vi "Get Bytes.vi"(11 "IMessagePackObject in":refnum<class "IMessagePackObject.lvclass">) -> (2 "Array":u8[](array[numeric]), 3 "IMessagePackObject out":refnum<class "IMessagePackObject.lvclass">)   [LabVIEW 2020, in "wamplv.lvlib" / "IMessagePackObject.lvclass"]
uses:
  IMessagePackObject.lvclass
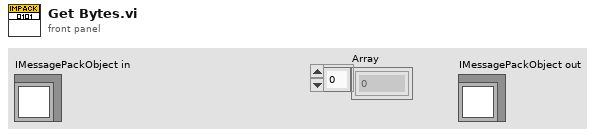
[diagram p1: front panel]
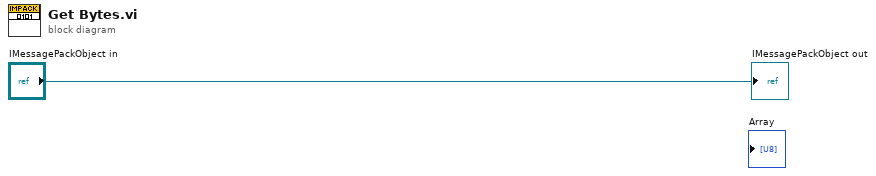
[diagram p0: block diagram]
diagram:
  "IMessagePackObject out" <- "IMessagePackObject in"
